vi "SwissSPAD Live_Clear Internal Variables.vi"(11 "SS2 Live Internal Variables in":T1={"okCFrontPanelDevices Refnum"=refnum, "Bottom Device Refnum"=refnum, "Display Image"=refnum, "# Live Images"=0, "relative s"=0.0, "# Image Sets"=0, "Message"="", "Current Image Set"=0, "# Datasets in Series"=0, "Current Dataset"=0, "Live Mode"=FALSE, "Recording Mode"=FALSE, "Record Button"=refnum, "\nLive Button"=refnum, "SwissSPAD Live Gate Image Data Q Name"="", "Discard First Image"=FALSE, "Image Information"={"Save ROI Only"=FALSE, "Left"=0, "Top"=0, "Right"=0, "Bottom"=0, "Use Current ROI"=FALSE}, "Image Binning Options"={"Use Image Binning"=FALSE, "X Bin"=0, "Y Bin"=0}, "Bottom FPGA Serial Number"="", "Detector PCB Version"=enum."SS2 PCB1", "# Acquisitions"=1, "10 bits"=FALSE, "Top FPGA Serial Number"="", "Top Device Refnum"=refnum} {"# Acquisitions" min=1; "Image Binning Options"."Y Bin" min=1; "Image Binning Options"."X Bin" min=1}) -> (3 "SS2 Live Internal Variables":T1={"okCFrontPanelDevices Refnum"=refnum, "Bottom Device Refnum"=refnum, "Display Image"=refnum, "# Live Images"=0, "relative s"=0.0, "# Image Sets"=0, "Message"="", "Current Image Set"=0, "# Datasets in Series"=0, "Current Dataset"=0, "Live Mode"=FALSE, "Recording Mode"=FALSE, "Record Button"=refnum, "\nLive Button"=refnum, "SwissSPAD Live Gate Image Data Q Name"="", "Discard First Image"=FALSE, "Image Information"={"Save ROI Only"=FALSE, "Left"=0, "Top"=0, "Right"=0, "Bottom"=0, "Use Current ROI"=FALSE}, "Image Binning Options"={"Use Image Binning"=FALSE, "X Bin"=0, "Y Bin"=0}, "Bottom FPGA Serial Number"="", "Detector PCB Version"=enum."SS2 PCB1", "# Acquisitions"=1, "10 bits"=FALSE, "Top FPGA Serial Number"="", "Top Device Refnum"=refnum} {"# Acquisitions" min=1; "Image Binning Options"."Y Bin" min=1; "Image Binning Options"."X Bin" min=1})   [LabVIEW 2021]
uses:
  SwissSPAD Live_Internal Variables.ctl
  D:/UCLA Thinkpad Google Drive/LabVIEW 2021 SP1/builds/SwissSPAD Live Distribution/Opal Kelly/C# Wrapper/v5.0.2/libFrontPanel-csharp.dll
  Opal Kelly/C# Wrapper/v5.0.2/libFrontPanel-csharp.dll
  <vilib>/vision/Image Controls.llb/IMAQ Image.ctl
  SwissSPAD Live_Image ROI Information.ctl
  Phasor/Image Binning Options.ctl
  SwissSPAD Live_SSx PCB Version.ctl
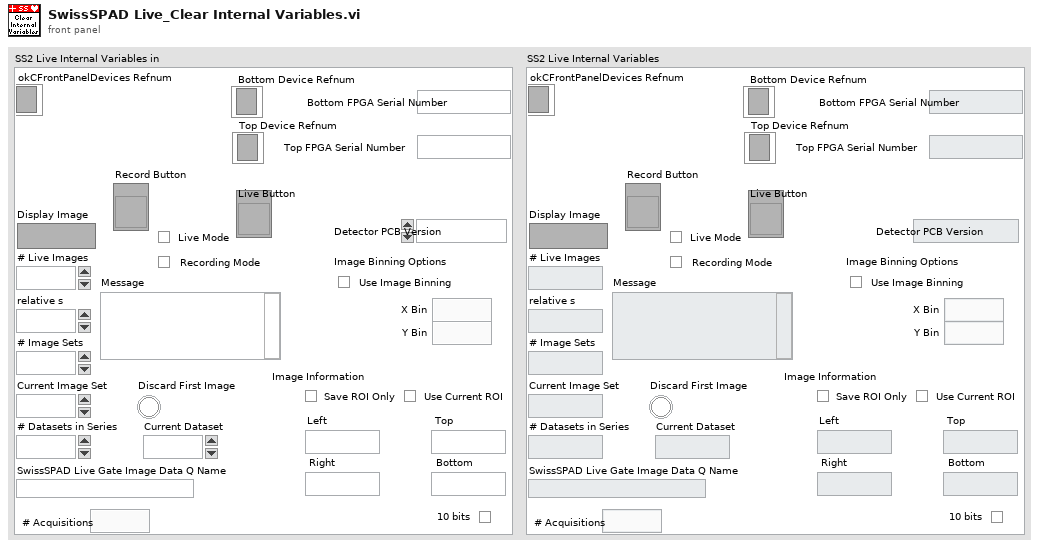
[diagram p1: front panel]
types:
  T1 = typedef "SwissSPAD Live_Internal Variables.ctl" = cluster{"okCFrontPanelDevices Refnum":refnum<k24>, "Bottom Device Refnum":refnum<k24>, "Display Image":T2, "# Live Images":i32, "relative s":dbl, "# Image Sets":i32, "Message":string, "Current Image Set":i32, "# Datasets in Series":i32, "Current Dataset":i32, "Live Mode":bool, "Recording Mode":bool, "Record Button":refnum<vi>, "\nLive Button":refnum<vi>, "SwissSPAD Live Gate Image Data Q Name":string, "Discard First Image":bool, "Image Information":T3, "Image Binning Options":T4, "Bottom FPGA Serial Number":string, "Detector PCB Version":T5, "# Acquisitions":u32, "10 bits":bool, "Top FPGA Serial Number":string, "Top Device Refnum":refnum<k24>}
  T2 = typedef "IMAQ Image.ctl" = refnum<image>
  T3 = typedef "SwissSPAD Live_Image ROI Information.ctl" = cluster{"Save ROI Only":bool, "Left":u16, "Top":u16, "Right":u16, "Bottom":u16, "Use Current ROI":bool}
  T4 = typedef "Image Binning Options.ctl" = cluster{"Use Image Binning":bool, "X Bin":i32, "Y Bin":i32}
  T5 = typedef "SwissSPAD Live_SSx PCB Version.ctl" = enum16{"unknown", "SS2 PCB1", "SS2 PCB2", "SS3 PCB1"}
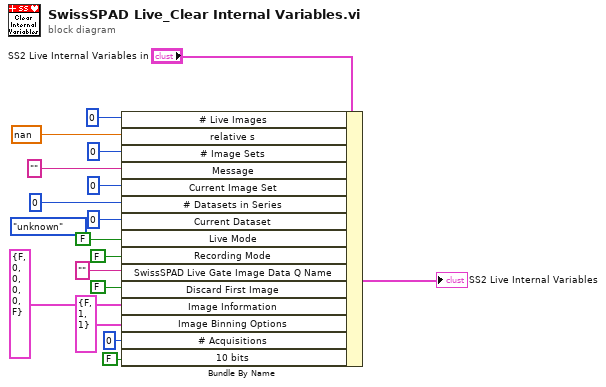
[diagram p0: block diagram]
diagram:
  (unwired) SwissSPAD_Live_SSx_PCB_Version."unknown" ("Detector PCB Version")
  n1 = Bundle By Name(cluster="SS2 Live Internal Variables in", "# Live Images"=0, "relative s"=nan, "# Image Sets"=0, "Message"="", "Current Image Set"=0, "# Datasets in Series"=0 ("# Datasets"), "Current Dataset"=0, "Live Mode"=FALSE, "Recording Mode"=FALSE, "SwissSPAD Live Gate Image Data Q Name"="" ("SS2 Live Gate Data Q Name"), "Discard First Image"=FALSE, "Image Information"=T3 {"Save ROI Only"=FALSE, "Left"=0, "Top"=0, "Right"=0, "Bottom"=0, "Use Current ROI"=FALSE}, "Image Binning Options"=T4 {"Use Image Binning"=FALSE, "X Bin"=1, "Y Bin"=1}, "# Acquisitions"=u32 0, "10 bits"=FALSE) -> (→"SS2 Live Internal Variables":T1)
